vi "Assign Instruments.vi"(8 "error in (no error)":errorcluster, 11 "Test Framework in":refnum<class "Test Framework.lvclass">) -> (0 "error out":errorcluster, 2 "Canceled":bool, 3 "Test Framework out":refnum<class "Test Framework.lvclass">)   [LabVIEW 2020, in "Test Framework.lvclass"]
doc: "Assigns the physical instruments to logical instruments for use in the test and which should be used as reference.\nOn load it will have the assigment from the last time the frame work ran.\nIn order to change assigment use the \"Search for Instruments\" button. This will update the found instrument list. Highlight the logical device and drag a found instrument into that location."
uses:
  Test Framework.lvclass
  Controls/Reference Selector.ctl
panel:
  in  "Clear Instrument Button":bool
  in  "Virtual Instruments":i32(listbox)
  in  "Instrument":string(combo)
  in  "Remove Button":bool
  in  "Add Button":bool
  in  "Clear Instruments Button":bool
  in  "Cancel Button":bool
  in  "Search Button":bool
  in  "10MHz Reference":T1
  in  "Instruments for tests":i32(listbox)
  in  "Found Instruments":i32(listbox)=-1
  in  "Done Button":bool
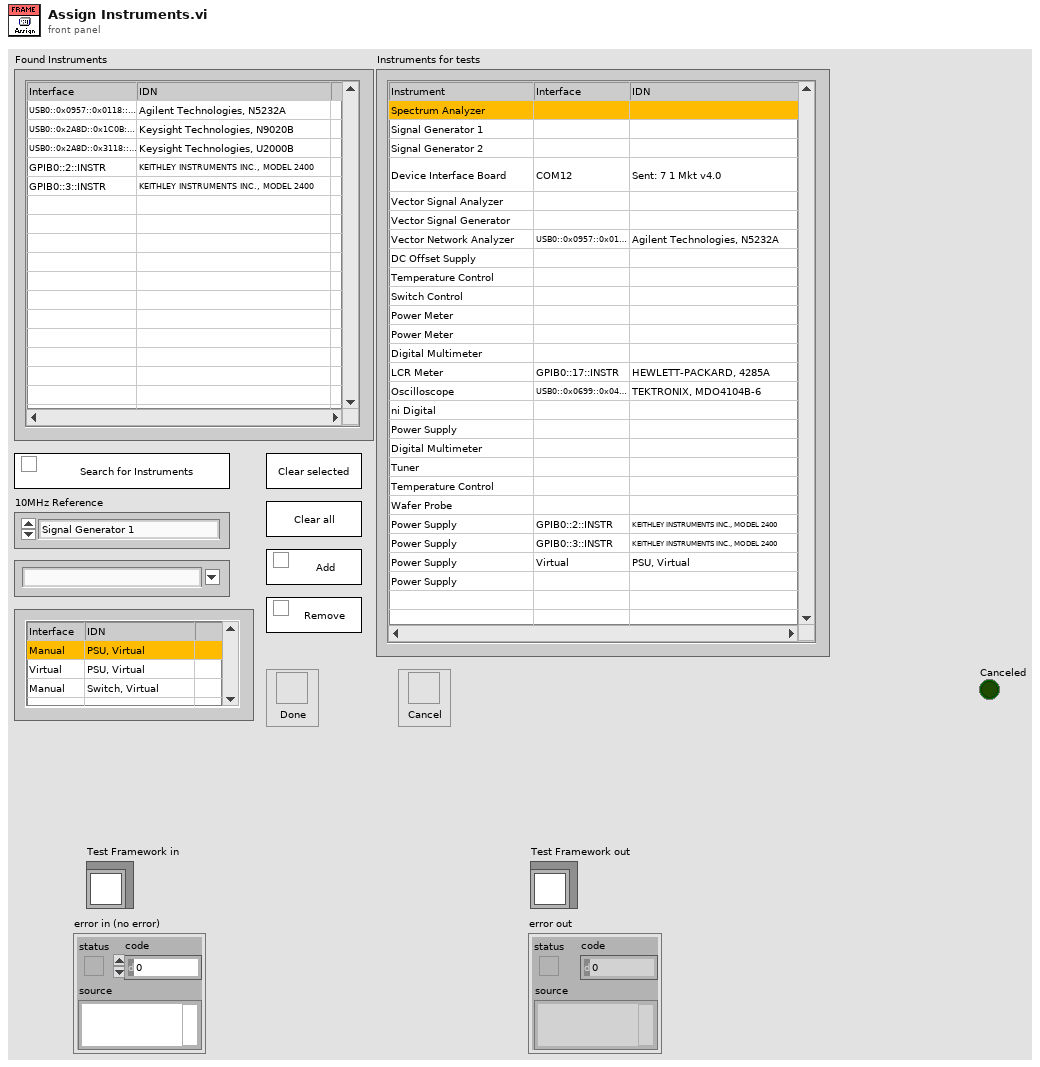
[diagram p1: front panel]
types:
  T1 = typedef "Test Framework.lvclass/Reference Selector.ctl" = enum16{"Signal Generator 1", "Signal Generator 2", "Spectrum Analyzer"}
  T2 = cluster{"Found Instruments":string[][], "Reference Selected":T1}
  T3 = cluster{"Found Instruments":bool[][], "Reference Selected":bool}
  T4 = cluster{"data name":string, "drag data":variant}[]
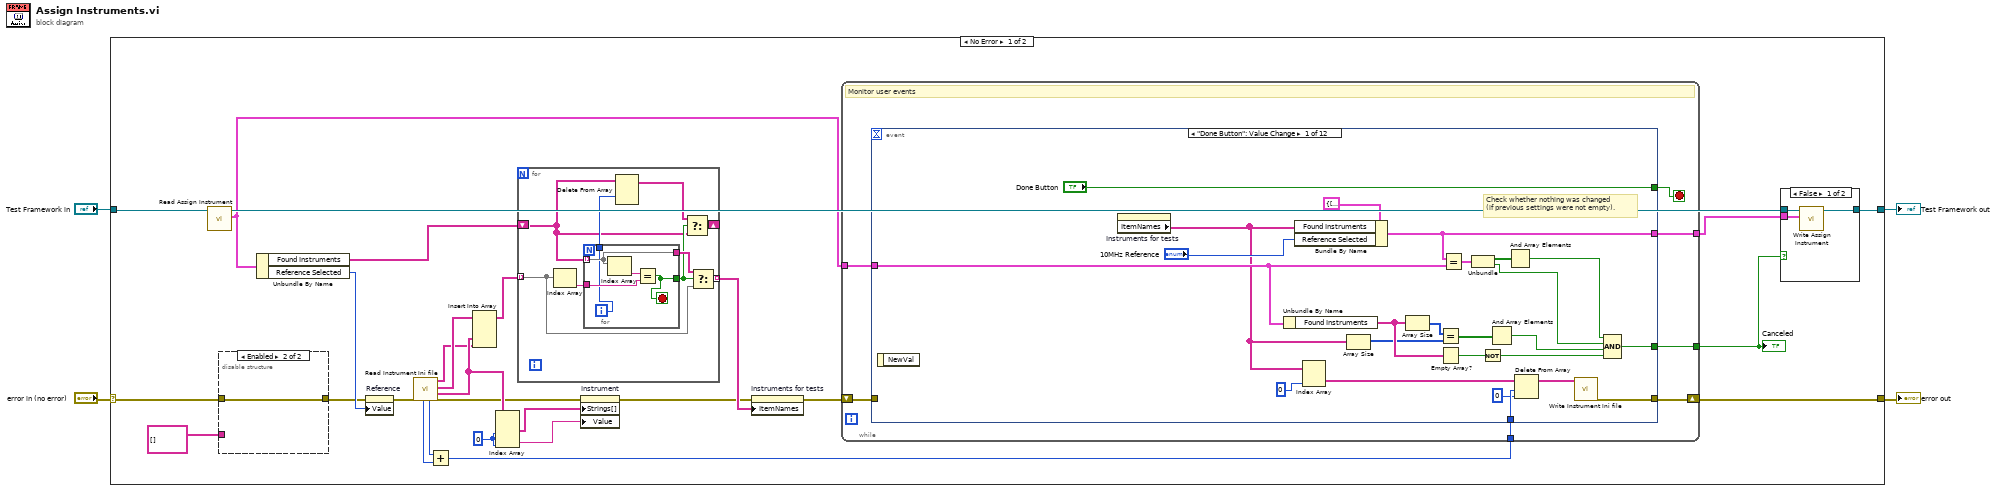
[diagram p0: block diagram]
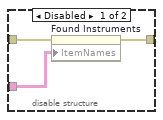
[diagram p2: hidden frame]
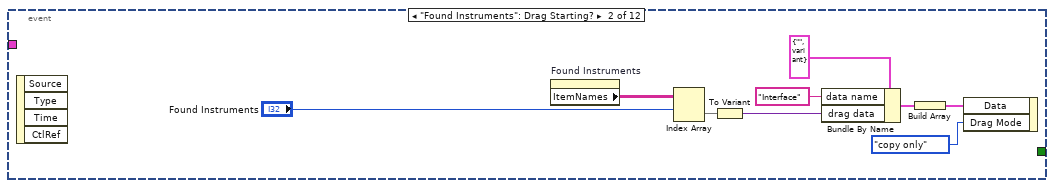
[diagram p4: hidden frame]
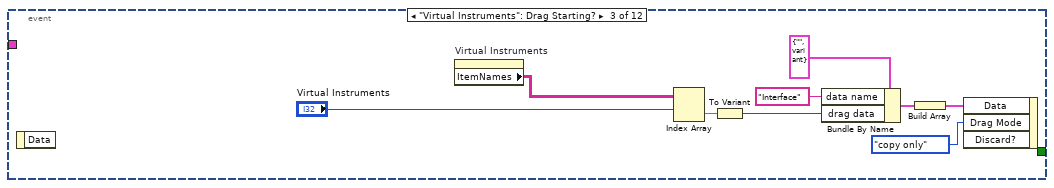
[diagram p5: hidden frame]
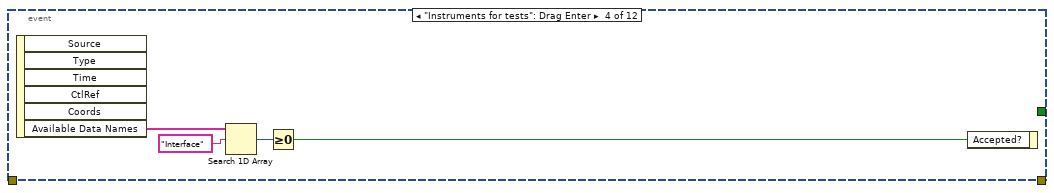
[diagram p6: hidden frame]
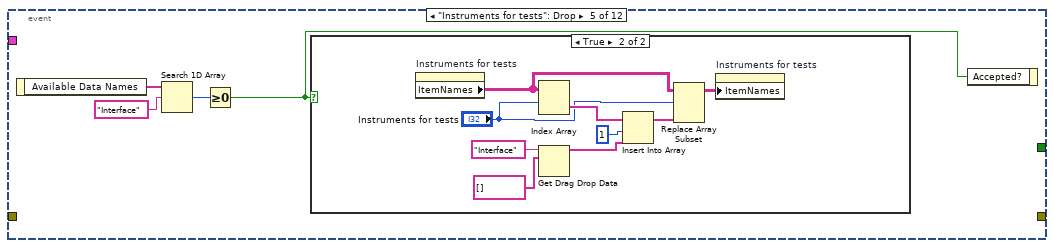
[diagram p7: hidden frame]
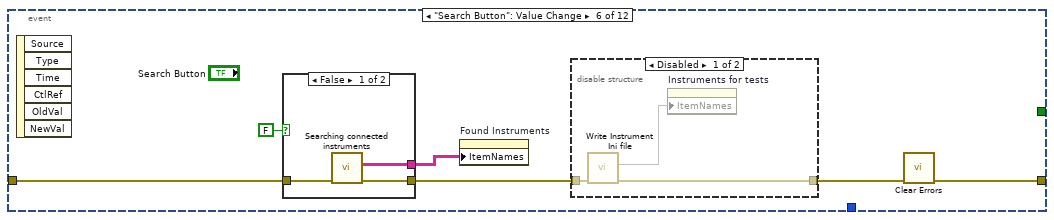
[diagram p9: hidden frame]
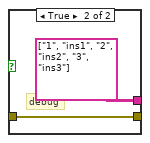
[diagram p10: hidden frame]
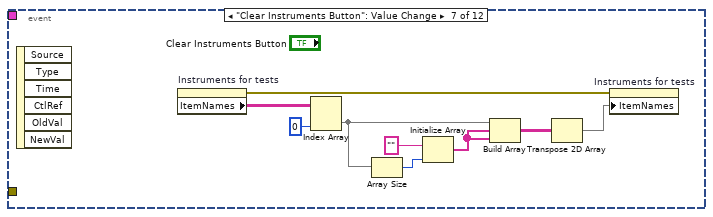
[diagram p12: hidden frame]
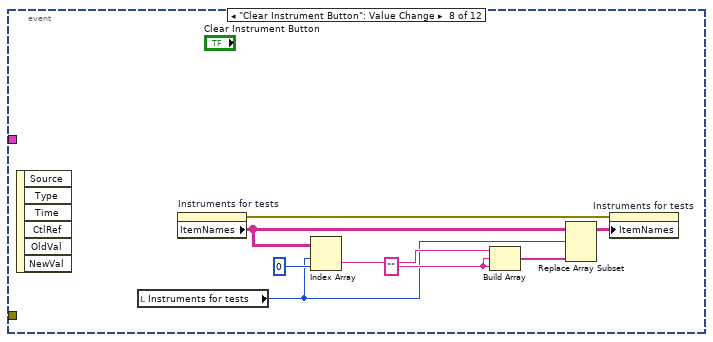
[diagram p13: hidden frame]
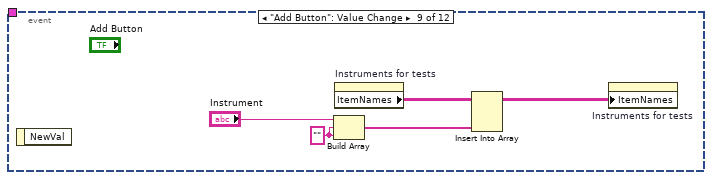
[diagram p14: hidden frame]
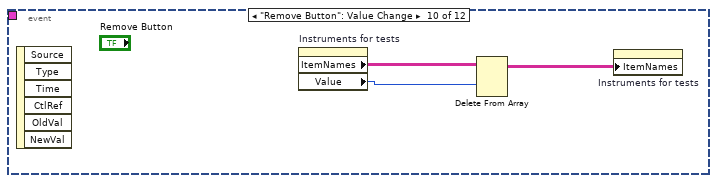
[diagram p15: hidden frame]
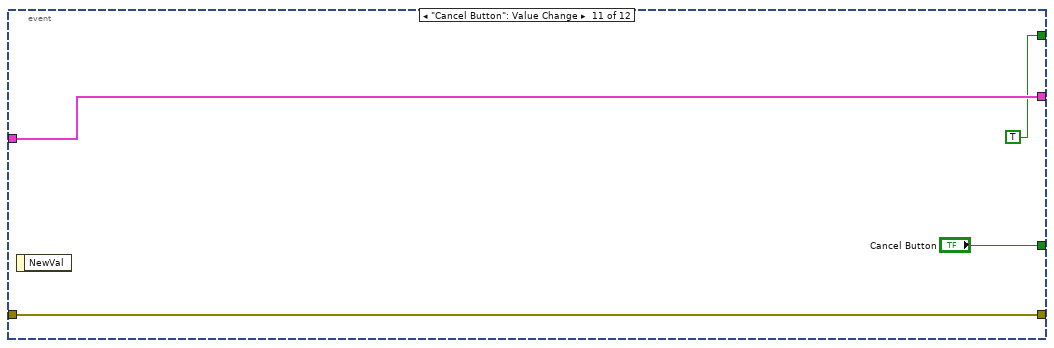
[diagram p16: hidden frame]
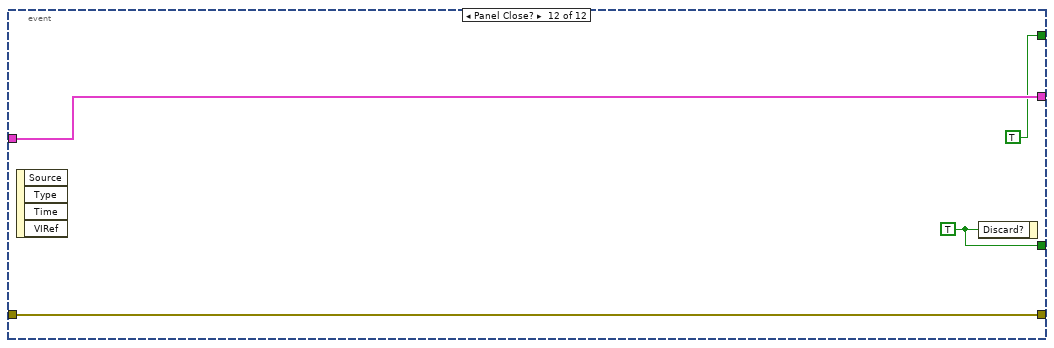
[diagram p17: hidden frame]
diagram:
  n1 = case shown="No Error" "error in (no error)" {
    selector: "error in (no error)" -> [w23 w169]
    tunnel: [w29 w168] -> w2
    tunnel: "Test Framework in" -> [w31 w168]
    tunnel: [w8 w169] -> w1
    frame No Error {
      w15 = 0 ("disabled index (col)")
      n2 = call-dynamic "Read Assign Instrument.vi"("Test Framework in"=w31) -> ("Assign Instrument"=w6:T2, "Test Framework out"=w30:refnum<class "Test Framework.lvclass">)  [unwired: 9 in]
      n3 = disable-structure shown="Enabled" {
        disable-tunnel: string[][] [] ("Item Names") -> [w34 _]
        disable-tunnel: w23 -> [w33 w35]
        disable-tunnel: [w32 w35] -> w22
        frame Disabled {
          n4 = property on="Found Instruments" class="MCListbox (strict)"(error in=w33, "ItemNames"=w34) -> (error out=w32:errorcluster)  [unwired: 1 in, 1 out]
        }
        frame Enabled {
        }
      }
      n5 = Unbundle By Name(w6) -> ("Found Instruments"=w25:string[][], "Reference Selected"=w26:T1)
      n6 = property on="Reference" class="Enum (strict)"(error in=w22, "Value"=w26) -> (error out=w27:errorcluster)  [unwired: 1 in, 1 out]
      n7 = call "Read Instrument Ini file.vi"("error in (no error)"=w27) -> ("error out"=w17:errorcluster, "Environmental List"=w19:string[][], "Instrument List"=w13:string[][], "User List"=w12:string[][], "# of Instruments"=w11:i32, "# of Environ"=w10:i32)  [unwired: 4 in, 1 out]
      n8 = Add(x=w11, y=w10) -> (x+y=w9:i32)
      n9 = Insert Into Array(array=w13, new element #1=w19, new element #2=w12) -> (w18:string[][])  [unwired: 2 in]
      n10 = Index Array(array=w19, index (col) #1=w15, index (row) #2=w15, index (col) #2=w15) -> (element #1=w20:string[], element #2=w14:string)  [unwired: 1 in]
      n11 = for {
        tunnel: w18 -> [w46] mode=indexing
        tunnel: [w45] -> w24 mode=indexing
        shift-right: [w43] -> _
        shift-left: w25 -> [w40]
        n12 = Index Array(array=w46) -> (element=w48:string)  [unwired: 1 in]
        n13 = for {
          tunnel: w40 -> [w53] mode=indexing
          tunnel: w48 -> [w51]
          tunnel: [w53] -> w47
          tunnel: [w50] -> w42
          tunnel: [w49] -> w44
          i -> [w49]
          stop <- w50 stop-if-true
          n14 = Index Array(array=w53) -> (element=w52:string)  [unwired: 1 in]
          n15 = Equal?(x=w52, y=w51) -> (x = y?=w50:bool)
        }
        n16 = Delete From Array(array=w40, index (row)=w44) -> (array with subset deleted=w41:string[][])  [unwired: 2 in, 1 out]
        n17 = Select(t=w41, s=w42, f=w40) -> (s? t:f=w43:string[][])
        n18 = Select(t=w47, s=w42, f=w46) -> (s? t:f=w45:string[])
      }
      n19 = property on="Instrument" class="CmbBox"(error in=w17, "Strings[]"=w20, "Value"=w14) -> (error out=w16:errorcluster)  [unwired: 1 in, 1 out]
      n20 = property on="Instruments for tests" class="MCListbox (strict)"(error in=w16, "ItemNames"=w24) -> (error out=w21:errorcluster)  [unwired: 1 in, 1 out]
      n21 = while {
        shift-right: [w55] -> w8
        shift-left: w21 -> [w59]
        tunnel: [w56] -> w7
        tunnel: w6 -> [w58]
        tunnel: w9 -> [w57]
        tunnel: [w54] -> w5
        stop <- w60 stop-if-true
        # "Monitor user events"
        n22 = event shown="[0] \"Done Button\": Value Change" {
          selector: _ -> [_ _ _ _ _ _ _ _ _ _ _ _]
          dyn-events: _ -> [_ _ _ _ _ _ _ _ _ _ _ _]
          timeout: _ -> [_ _ _ _ _ _ _ _ _ _ _ _]
          tunnel: ["Done Button" _ _ _ _ _ _ _ _ _ TRUE ("Done Button") TRUE ("Done Button")] -> w60
          tunnel: w59 -> [_ _ _ _ _ w125 _ _ _ _ w161 w165]
          tunnel: [w76 _ _ _ _ w120 _ _ _ _ w161 w165] -> w55
          tunnel: [w72 _ _ _ _ _ _ _ _ _ w163 w167] -> w56
          tunnel: w58 -> [w71 _ _ _ _ _ _ _ _ _ w163 w167]
          tunnel: w57 -> [w78 _ _ _ _ _ _ _ _ _ _ _]
          tunnel: [w61 _ _ _ _ _ _ _ _ _ "Cancel Button" w164] -> w54
          event "Done Button": Value Change {
            # "Check whether nothing was changed \n(if previous settings were not empty)."
            n23 = event-data() -> ()  [unwired: 1 in, 1 out]
            n24 = property on="Instruments for tests" class="MCListbox (strict)"() -> ("ItemNames"=w67:string[][])  [unwired: 2 in, 2 out]
            n25 = Unbundle By Name(w71) -> ("Found Instruments"=w68:string[][])
            n26 = Bundle By Name(cluster=T2 {"Found Instruments"=[], "Reference Selected"=enum."Signal Generator 1"} ("Assign Instrument"), "Found Instruments"=w67, "Reference Selected"="10MHz Reference") -> (w72:T2)
            n27 = Index Array(array=w67, index (col)=0 ("disabled index (col)")) -> (element=w81:string[])  [unwired: 1 in]
            n28 = Array Size(array=w67) -> (size(s)=w65:i32[])
            n29 = Array Size(array=w68) -> (size(s)=w66:i32[])
            n30 = Equal?(x=w66, y=w65) -> (x = y?=w64:bool[])
            n31 = Empty Array?(array=w68) -> (empty?=w69:bool)
            n32 = Equal?(x=w72, y=w71) -> (x = y?=w75:T3)
            n33 = Unbundle(w75) -> ("Found Instruments"=w74:bool[][], "Reference Selected"=w70:bool)
            n34 = Not(x=w69) -> (.not. x?=w62:bool)
            n35 = And Array Elements(Boolean array=w64) -> (logical AND=w63:bool)
            n36 = And Array Elements(Boolean array=w74) -> (logical AND=w73:bool)
            n37 = Delete From Array(array=w81, length=w78, index=0) -> (array with subset deleted=w80:string[])  [unwired: 1 out]
            n38 = call "Write Instrument Ini file.vi"("User List"=w80) -> ("error out"=w76:errorcluster)  [unwired: 10 in]
            n39 = Compound Arithmetic op=AND(w73, w70, w63, w62) -> (w61:bool)
          }
          event "Found Instruments": Drag Starting? {
            n40 = event-data() -> ()  [unwired: 1 in, 4 out]
            n41 = property on="Found Instruments" class="MCListbox (strict)"() -> ("ItemNames"=w93:string[][])  [unwired: 2 in, 2 out]
            n42 = Index Array(array=w93, index (row)="Found Instruments") -> (element=w88:string[])  [unwired: 1 in]
            n43 = To Variant(anything=w88) -> (Variant=w89:variant)
            n44 = Bundle By Name(cluster=cluster{"data name":string, "drag data":variant} {"data name"="", "drag data"=variant}, "data name"="Interface", "drag data"=w89) -> (w87:cluster{"data name":string, "drag data":variant})
            n45 = Build Array(w87) -> (w86:T4)
            n46 = event-data("Data"=w86, "Drag Mode"=enum32{"copy or move", "copy only", "move only"}."copy only") -> ()  [unwired: 1 in, 1 out]
          }
          event "Virtual Instruments": Drag Starting? {
            n47 = event-data() -> ()  [unwired: 1 in, 1 out]
            n48 = property on="Virtual Instruments" class="MCListbox (strict)"() -> ("ItemNames"=w95:string[][])  [unwired: 2 in, 2 out]
            n49 = Index Array(array=w95, index (row)="Virtual Instruments") -> (element=w99:string[])  [unwired: 1 in]
            n50 = To Variant(anything=w99) -> (Variant=w100:variant)
            n51 = Bundle By Name(cluster=cluster{"data name":string, "drag data":variant} {"data name"="", "drag data"=variant}, "data name"="Interface", "drag data"=w100) -> (w98:cluster{"data name":string, "drag data":variant})
            n52 = Build Array(w98) -> (w97:T4)
            n53 = event-data("Data"=w97, "Drag Mode"=enum32{"copy or move", "copy only", "move only"}."copy only") -> ()  [unwired: 2 in, 1 out]
          }
          event "Instruments for tests": Drag Enter {
            n54 = event-data() -> ("Available Data Names"=w106:string[])  [unwired: 1 in, 5 out]
            n55 = Search 1D Array(1D array=w106, element="Interface" ("data name")) -> (index of element=w104:i32)  [unwired: 1 in]
            n56 = Greater Or Equal To 0?(x=w104) -> (x >= 0?=w103:bool)
            n57 = event-data("Accepted?"=w103) -> ()  [unwired: 1 in, 1 out]
          }
          event "Instruments for tests": Drop {
            n58 = event-data() -> ("Available Data Names"=w108:string[])  [unwired: 1 in]
            n59 = Search 1D Array(1D array=w108, element="Interface" ("data name")) -> (index of element=w109:i32)  [unwired: 1 in]
            n60 = Greater Or Equal To 0?(x=w109) -> (x >= 0?=w107:bool)
            n61 = case shown="True" w107 {
              frame False {
              }
              frame True {
                n62 = property on="Instruments for tests" class="MCListbox (strict)"() -> ("ItemNames"=w116:string[][])  [unwired: 2 in, 2 out]
                n63 = Index Array(array=w116, index (row)="Instruments for tests") -> (element=w115:string[])  [unwired: 1 in]
                n64 = Get Drag Drop Data(8:string[] [], 9:"Interface" ("data name")) -> (3:w114:string[])  [unwired: 1 in, 1 out]
                n65 = Insert Into Array(array=w115, index=1, new element=w114) -> (w113:string[])
                n66 = Replace Array Subset(array=w116, new element=w113, index (row)="Instruments for tests") -> (w117:string[][])  [unwired: 1 in]
                n67 = property on="Instruments for tests" class="MCListbox (strict)"("ItemNames"=w117) -> ()  [unwired: 2 in, 2 out]
              }
            }
            n68 = event-data("Accepted?"=w107) -> ()  [unwired: 1 in, 1 out]
          }
          event "Search Button": Value Change {
            n69 = event-data() -> ()  [unwired: 1 in, 6 out]
            n70 = case shown="False" FALSE {
              tunnel: w125 -> [w128 w130]
              tunnel: [w127 string[][] [["1", "ins1"], ["2", "ins2"], ["3", "ins3"]] ("Found Instruments")] -> w124
              tunnel: [w126 w130] -> w123
              frame False {
                n71 = call "Searching connected instruments.vi"("error in (no error)"=w128) -> ("error out"=w126:errorcluster, "Found Instruments"=w127:string[][])  [unwired: 9 in]
              }
              frame True {
                # "debug"
              }
            }
            n72 = property on="Found Instruments" class="MCListbox (strict)"("ItemNames"=w124) -> ()  [unwired: 2 in, 2 out]
            n73 = disable-structure shown="Disabled" {
              disable-tunnel: w123 -> [w133 w134]
              disable-tunnel: [w132 w134] -> w121
              frame Disabled {
                n74 = call "Write Instrument Ini file.vi"("error in (no error)"=w133) -> ("error out"=w132:errorcluster, 2:w131)  [unwired: 9 in]
                n75 = property on="Instruments for tests" class="MCListbox (strict)"("ItemNames"=w131) -> ()  [unwired: 2 in, 2 out]
              }
              frame Enabled {
              }
            }
            n76 = call <vilib>:"Clear Errors.vi"("error in (no error)"=w121) -> ("error out"=w120:errorcluster)  [unwired: 5 in, 1 out]
          }
          event "Clear Instruments Button": Value Change {
            n77 = event-data() -> ()  [unwired: 1 in, 6 out]
            n78 = property on="Instruments for tests" class="MCListbox (strict)"() -> (error out=w143:errorcluster, "ItemNames"=w141:string[][])  [unwired: 2 in, 1 out]
            n79 = Index Array(array=w141, index (col)=0 ("disabled index (col)")) -> (element=w139:string[])  [unwired: 1 in]
            n80 = Array Size(array=w139) -> (size(s)=w140:i32)
            n81 = Initialize Array("", w140) -> (w138:string[])
            n82 = Build Array(w139, w138, w138) -> (w136:string[][])
            n83 = Transpose 2D Array(2D array=w136) -> (transposed array=w135:string[][])
            n84 = property on="Instruments for tests" class="MCListbox (strict)"(error in=w143, "ItemNames"=w135) -> ()  [unwired: 1 in, 2 out]
          }
          event "Clear Instrument Button": Value Change {
            w149 = ""
            n85 = event-data() -> ()  [unwired: 1 in, 6 out]
            n86 = local read "Instruments for tests"() -> (w146:i32)
            n87 = property on="Instruments for tests" class="MCListbox (strict)"() -> (error out=w151:errorcluster, "ItemNames"=w147:string[][])  [unwired: 2 in, 1 out]
            n88 = Index Array(array=w147, index (row)=w146, index (col)=0 ("disabled index (col)")) -> (element=w150:string)
            n89 = Build Array(w150, w149, w149) -> (w145:string[])
            n90 = Replace Array Subset(array=w147, new element=w145, index (row)=w146) -> (w144:string[][])  [unwired: 1 in]
            n91 = property on="Instruments for tests" class="MCListbox (strict)"(error in=w151, "ItemNames"=w144) -> ()  [unwired: 1 in, 2 out]
          }
          event "Add Button": Value Change {
            w152 = "" ("element")
            n92 = event-data() -> ()  [unwired: 1 in, 1 out]
            n93 = Build Array("Instrument", w152, w152) -> (w153:string[])
            n94 = property on="Instruments for tests" class="MCListbox (strict)"() -> ("ItemNames"=w156:string[][])  [unwired: 2 in, 2 out]
            n95 = Insert Into Array(array=w156, new element=w153) -> (w155:string[][])  [unwired: 2 in]
            n96 = property on="Instruments for tests" class="MCListbox (strict)"("ItemNames"=w155) -> ()  [unwired: 2 in, 2 out]
          }
          event "Remove Button": Value Change {
            n97 = event-data() -> ()  [unwired: 1 in, 6 out]
            n98 = property on="Instruments for tests" class="MCListbox (strict)"() -> ("ItemNames"=w159:string[][], "Value"=w157:i32)  [unwired: 2 in, 2 out]
            n99 = Delete From Array(array=w159, index (row)=w157) -> (array with subset deleted=w158:string[][])  [unwired: 2 in, 1 out]
            n100 = property on="Instruments for tests" class="MCListbox (strict)"("ItemNames"=w158) -> ()  [unwired: 2 in, 2 out]
          }
          event "Cancel Button": Value Change {
            n101 = event-data() -> ()  [unwired: 1 in, 1 out]
          }
          event Panel Close? {
            w164 = TRUE
            n102 = event-data() -> ()  [unwired: 1 in, 4 out]
            n103 = event-data("Discard?"=w164) -> ()  [unwired: 1 in, 1 out]
          }
        }
      }
      "Canceled" <- w5
      n104 = case shown="False" w5 {
        tunnel: w30 -> [w38 w39]
        tunnel: [w37 w39] -> w29
        tunnel: w7 -> [w36 _]
        frame False {
          n105 = call-dynamic "Write Assign Instrument.vi"("Assign Instrument"=w36, "Test Framework in"=w38) -> ("Test Framework out"=w37:refnum<class "Test Framework.lvclass">)  [unwired: 9 in]
        }
        frame True {
        }
      }
    }
    frame Error {
    }
  }
  "error out" <- w1
  "Test Framework out" <- w2
